vi "Finish.vi"   [LabVIEW 2012]
doc: "This VI is called just before exiting. It is expected to close I/O refnum, save collected data, etc."
uses:
  <vilib>/Rock Robotics/WPI/Joystick/WPI_JoystickGetSetRefNum.vi
  <vilib>/Rock Robotics/WPI/Compressor/WPI_CompressorGetSetRefNum.vi
  <vilib>/Rock Robotics/WPI/RobotDrive/WPI_RobotDriveGetSetRefNum.vi
types:
  T1 = typedef "WPI_MotorControlDeviceRef.ctl" = cluster{"DeviceStatus":errorcluster, "Type":enum16{"PWM", "CAN"}, "PWM":cluster{"Digital Module":T2, "PWM Channel":T3, "DeadBand":T4}, "CAN":cluster{"Device Number":u8, "Control Mode":T5, "Semaphore":T6, "Max Vout":dbl}, "Invert":bool, "TransformRef":T7, "InvTransformRef":T7}
  T2 = typedef "FPGA_TypedefDigitalModule.ctl" = enum16{"Digital Module 1", "Digital Module 2"}
  T3 = typedef "FPGA_DIOPWMChannel.ctl" = enum8{"PWM 1", "PWM 2", "PWM 3", "PWM 4", "PWM 5", "PWM 6", "PWM 7", "PWM 8", "PWM 9", "PWM 10", "Invalid"}
  T4 = typedef "WPI_PWMDeadband.ctl" = cluster{"Name":string, "maxPositivePwm":i32, "minPositivePwm":i32, "centerPwm":i32, "maxNegativePwm":i32, "minNegativePwm":i32, "angularRange":u16}
  T5 = typedef "WPI_CANJaguar_ControlMode.ctl" = enum8{"Percent VBus", "Current", "Speed", "Position", "Voltage"}
  T6 = typedef "Semaphore RefNum" = refnum<k1>
  T7 = typedef "WPI_PWMTransform_ConPane.ctl" = refnum<vi>
  T8 = typedef "WPI_RobotDriveDevRef.ctl" = cluster{"DevStatus":errorcluster, "Motors[]":T1[], "Square Inputs":bool, "Max Output":dbl, "Isochronous":bool}
  T9 = typedef "WPI_JoystickDevRef.ctl" = cluster{"Device":T10}
  T10 = typedef "WPI_JoystickDeviceEnum.ctl" = enum16{"USB 1", "USB 2", "USB 3", "USB 4", "Kinect 1", "Kinect 2"}
  T11 = typedef "WPI_DigitalInputDevRef.ctl" = cluster{"DevStatus":errorcluster, "DIO Channel":T12, "Digital Module":T2}
  T12 = typedef "FPGA_DIOChannel.ctl" = enum8{"DIO 1", "DIO 2", "DIO 3", "DIO 4", "DIO 5", "DIO 6", "DIO 7", "DIO 8", "DIO 9", "DIO 10", "DIO 11", "DIO 12", "DIO 13", "DIO 14", "Invalid"}
  T13 = typedef "WPI_AnalogChannelDevRef.ctl" = cluster{"DevStatus":errorcluster, "Analog Module":T14, "Analog Channel":T15}
  T14 = typedef "FPGA_TypedefAnalogModule.ctl" = enum16{"Analog Module 1", "Analog Module 2"}
  T15 = typedef "FPGA_AIChannel.ctl" = enum8{"AI 1", "AI 2", "AI 3", "AI 4", "AI 5", "AI 6", "AI 7", "AI 8", "Invalid"}
  T16 = typedef "WPI_CompressorDevRef.ctl" = cluster{"DevStatus":errorcluster, "DigitalInputDevRef":T11, "RelayDevRef":T17}
  T17 = typedef "WPI_RelayDevRef.ctl" = cluster{"DevStatus":errorcluster, "Relay Channel":T18, "Digital Module":T2, "Relay Direction":T19}
  T18 = typedef "FPGA_DIORelayChannel.ctl" = enum8{"Relay 1", "Relay 2", "Relay 3", "Relay 4", "Relay 5", "Relay 6", "Relay 7", "Relay 8", "Invalid"}
  T19 = typedef "WPI_RelayDirection.ctl" = enum16{"Both directions", "Forward only", "Reverse only"}
  T20 = typedef "WPI_CameraDevRef.ctl" = cluster{"Camera Address":string, "CameraStatus":errorcluster, "Acquire Image Notifier":refnum<notifier>}
  T21 = typedef "WPI_SolenoidDevRef.ctl" = cluster{"DevStatus":errorcluster, "Solenoid Module":T22, "Forward Solenoid Channel":T23, "Reverse Solenoid Channel":T23}
  T22 = typedef "FPGA_TypedefSolenoidModule.ctl" = enum16{"Solenoid Module 1", "Solenoid Module 2"}
  T23 = typedef "WPI_SolenoidChannel.ctl" = enum8{"Solenoid 1", "Solenoid 2", "Solenoid 3", "Solenoid 4", "Solenoid 5", "Solenoid 6", "Solenoid 7", "Solenoid 8", "Invalid"}
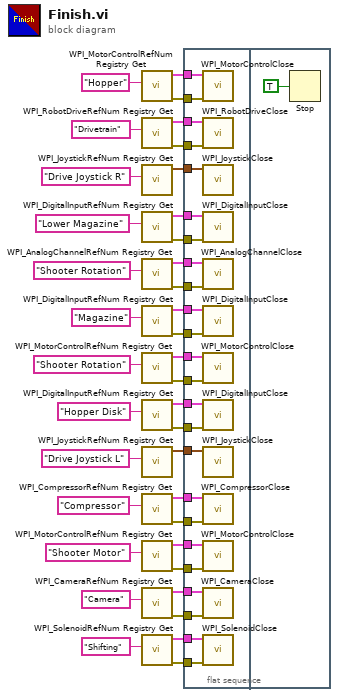
[diagram p0: block diagram]
diagram:
  n1 = call <vilib>:"WPI_MotorControlRefNum Registry Get.vi"("refnum name"="Hopper") -> ("error out"=w6:errorcluster, "MotorControlDevRef"=w7:T1)  [unwired: 9 in]
  n2 = call <vilib>:"WPI_RobotDriveRefNum Registry Get.vi"("refnum name"="Drivetrain") -> ("error out"=w23:errorcluster, "RobotDriveDevRef"=w36:T8)  [unwired: 1 in, 8 out]
  n3 = call <vilib>:"WPI_JoystickRefNum Registry Get.vi"("refnum name"="Drive Joystick R") -> ("JoystickDevRef"=w25:T9)  [unwired: 1 in, 9 out]
  n4 = call <vilib>:"WPI_DigitalInputRefNum Registry Get.vi"("refnum name"="Lower Magazine") -> ("error out"=w13:errorcluster, "DigitalInputDevRef"=w14:T11)  [unwired: 9 in]
  n5 = call <vilib>:"WPI_AnalogChannelRefNum Registry Get.vi"("refnum name"="Shooter Rotation") -> ("error out"=w11:errorcluster, "AIDeviceRef"=w12:T13)  [unwired: 9 in]
  n6 = call <vilib>:"WPI_DigitalInputRefNum Registry Get.vi"("refnum name"="Magazine") -> ("error out"=w15:errorcluster, "DigitalInputDevRef"=w16:T11)  [unwired: 9 in]
  n7 = call <vilib>:"WPI_MotorControlRefNum Registry Get.vi"("refnum name"="Shooter Rotation") -> ("error out"=w8:errorcluster, "MotorControlDevRef"=w9:T1)  [unwired: 9 in]
  n8 = call <vilib>:"WPI_DigitalInputRefNum Registry Get.vi"("refnum name"="Hopper Disk") -> ("error out"=w17:errorcluster, "DigitalInputDevRef"=w18:T11)  [unwired: 9 in]
  n9 = call <vilib>:"WPI_JoystickRefNum Registry Get.vi"("refnum name"="Drive Joystick L") -> ("JoystickDevRef"=w24:T9)  [unwired: 1 in, 9 out]
  n10 = call <vilib>:"WPI_CompressorRefNum Registry Get.vi"("refnum name"="Compressor") -> ("error out"=w29:errorcluster, "CompressorDevRef"=w30:T16)  [unwired: 9 in]
  n11 = call <vilib>:"WPI_MotorControlRefNum Registry Get.vi"("refnum name"="Shooter Motor") -> ("error out"=w4:errorcluster, "MotorControlDevRef"=w5:T1)  [unwired: 9 in]
  n12 = call <vilib>:"WPI_CameraRefNum Registry Get.vi"("refnum name"="Camera") -> ("error out"=w22:errorcluster, "CameraDevRef"=w35:T20)  [unwired: 1 in, 8 out]
  n13 = call <vilib>:"WPI_SolenoidRefNum Registry Get.vi"("refnum name"="Shifting") -> ("error out"=w31:errorcluster, "SolenoidDevRef"=w32:T21)  [unwired: 9 in]
  n14 = flat-sequence {
    tunnel: w36 -> [w61]
    tunnel: w35 -> [w60]
    tunnel: w32 -> [w59]
    tunnel: w31 -> [w58]
    tunnel: w30 -> [w57]
    tunnel: w29 -> [w56]
    tunnel: w25 -> [w55]
    tunnel: w24 -> [w54]
    tunnel: w23 -> [w53]
    tunnel: w22 -> [w52]
    tunnel: w18 -> [w51]
    tunnel: w17 -> [w50]
    tunnel: w16 -> [w49]
    tunnel: w15 -> [w48]
    tunnel: w14 -> [w47]
    tunnel: w13 -> [w46]
    tunnel: w12 -> [w45]
    tunnel: w11 -> [w44]
    tunnel: w9 -> [w43]
    tunnel: w8 -> [w42]
    tunnel: w7 -> [w41]
    tunnel: w6 -> [w40]
    tunnel: w5 -> [w39]
    tunnel: w4 -> [w38]
    frame #0 {
      n15 = call <vilib>:"WPI_MotorControlClose.vi"("error in (no error)"=w40, "MotorControlDevRef"=w41) -> ()  [unwired: 9 in, 1 out]
      n16 = call <vilib>:"WPI_RobotDriveClose.vi"("error in (no error)"=w53, "RobotDriveDevRef"=w61) -> ()  [unwired: 10 out]
      n17 = call <vilib>:"WPI_JoystickClose.vi"("JoystickDevRef"=w55) -> ()  [unwired: 11 out]
      n18 = call <vilib>:"WPI_DigitalInputClose.vi"("error in (no error)"=w46, "DigitalInputDevRef"=w47) -> ()  [unwired: 9 in, 1 out]
      n19 = call <vilib>:"WPI_AnalogChannelClose.vi"("error in (no error)"=w44, "AIDeviceRef"=w45) -> ()  [unwired: 9 in, 1 out]
      n20 = call <vilib>:"WPI_DigitalInputClose.vi"("error in (no error)"=w48, "DigitalInputDevRef"=w49) -> ()  [unwired: 9 in, 1 out]
      n21 = call <vilib>:"WPI_MotorControlClose.vi"("error in (no error)"=w42, "MotorControlDevRef"=w43) -> ()  [unwired: 9 in, 1 out]
      n22 = call <vilib>:"WPI_DigitalInputClose.vi"("error in (no error)"=w50, "DigitalInputDevRef"=w51) -> ()  [unwired: 9 in, 1 out]
      n23 = call <vilib>:"WPI_JoystickClose.vi"("JoystickDevRef"=w54) -> ()  [unwired: 11 out]
      n24 = call <vilib>:"WPI_CompressorClose.vi"("error in (no error)"=w56, "CompressorDevRef"=w57) -> ()  [unwired: 9 in, 1 out]
      n25 = call <vilib>:"WPI_MotorControlClose.vi"("error in (no error)"=w38, "MotorControlDevRef"=w39) -> ()  [unwired: 9 in, 1 out]
      n26 = call <vilib>:"WPI_CameraClose.vi"("error in (no error)"=w52, "CameraDevRef"=w60) -> ()  [unwired: 10 out]
      n27 = call <vilib>:"WPI_SolenoidClose.vi"("error in (no error)"=w58, "SolenoidDevRef"=w59) -> ()  [unwired: 9 in, 1 out]
    }
    frame #1 {
      n28 = Stop(stop? (T)=TRUE ("Quit")) -> ()
    }
  }
